vi "Read Supported Protocols.vi"(8 "error in (no error)":errorcluster, 11 "Connection.WS in":refnum<class "Connection.WS.lvclass">) -> (0 "error out":errorcluster, 1 "All?":bool, 2 "Supported Protocols":string[](array[string]), 3 "Connection.WS out":refnum<class "Connection.WS.lvclass">)   [LabVIEW 2013, in "Connection.WS_GOSPL.lvlib" / "Connection.WS.lvclass"]
uses:
  Connection.WS.lvclass
  Connection.WS.lvclass/Connection.WS.ctl
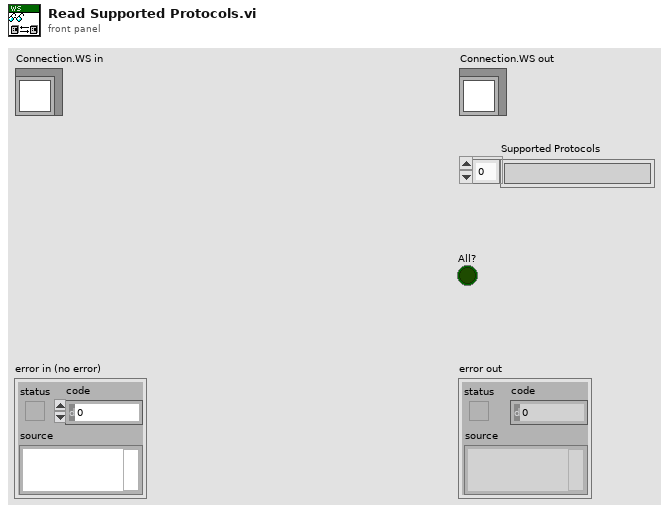
[diagram p1: front panel]
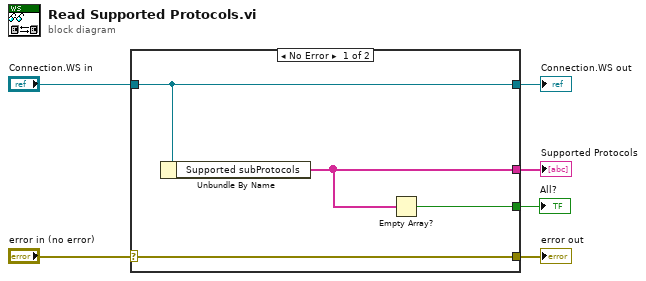
[diagram p0: block diagram]
diagram:
  n1 = case shown="No Error" "error in (no error)" {
    selector: "error in (no error)" -> [w10 w11]
    tunnel: [w10 w11] -> w5
    tunnel: [w9 w12] -> w3
    tunnel: "Connection.WS in" -> [w9 w12]
    tunnel: [w8 _] -> w2
    tunnel: [w7 _] -> w1
    frame No Error {
      n2 = Unbundle By Name(w9) -> ("Supported subProtocols"=w8:string[])
      n3 = Empty Array?(array=w8) -> (empty?=w7:bool)
    }
    frame Error {
    }
  }
  "error out" <- w5
  "Connection.WS out" <- w3
  "Supported Protocols" <- w2
  "All?" <- w1
